vi "Histogram Main.vi"() -> ()   [LabVIEW 2012]
uses:
  Consumer Message.ctl
  <vilib>/Utility/file.llb/Write To Spreadsheet File (DBL).vi
panel:
  in  "signal":u16(ring) items=["uniform white", "uniform+uniform", "Gaussian white", "sine", "square"]
  in  "Snapshot":bool
  out "Histogram":cluster{"histogram":dbl[], "x axis":dbl[]}(graph)
  in  "bins":i32=20
  out "Consumer Shutdown?":bool
  out "Backlog":u8(slide) scale=0.0..100.0
  in  "Stop":bool
  # "Number of enqueued messages waiting to be processed"
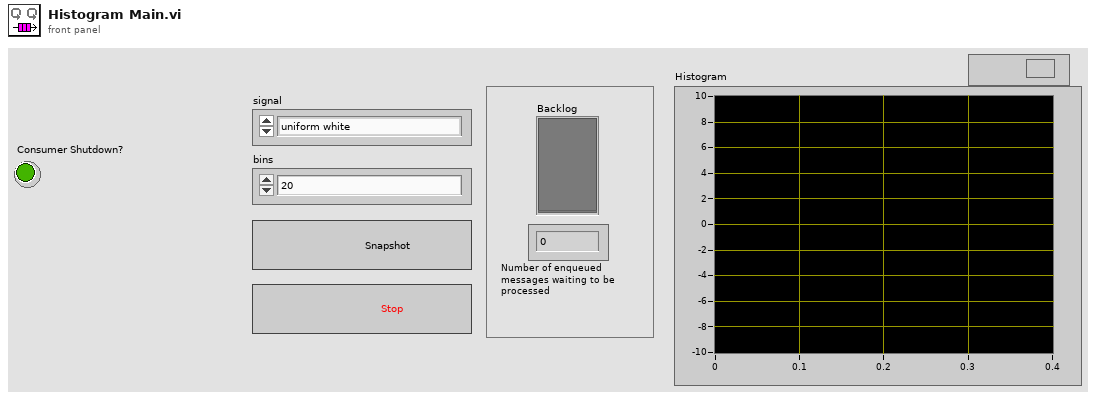
[diagram p1: front panel]
types:
  T1 = typedef "Consumer Message.ctl" = cluster{"Consumer State":string, "Boolean Data":bool, "Numeric Data":i32, "Signal":dbl[], "Error":errorcluster}
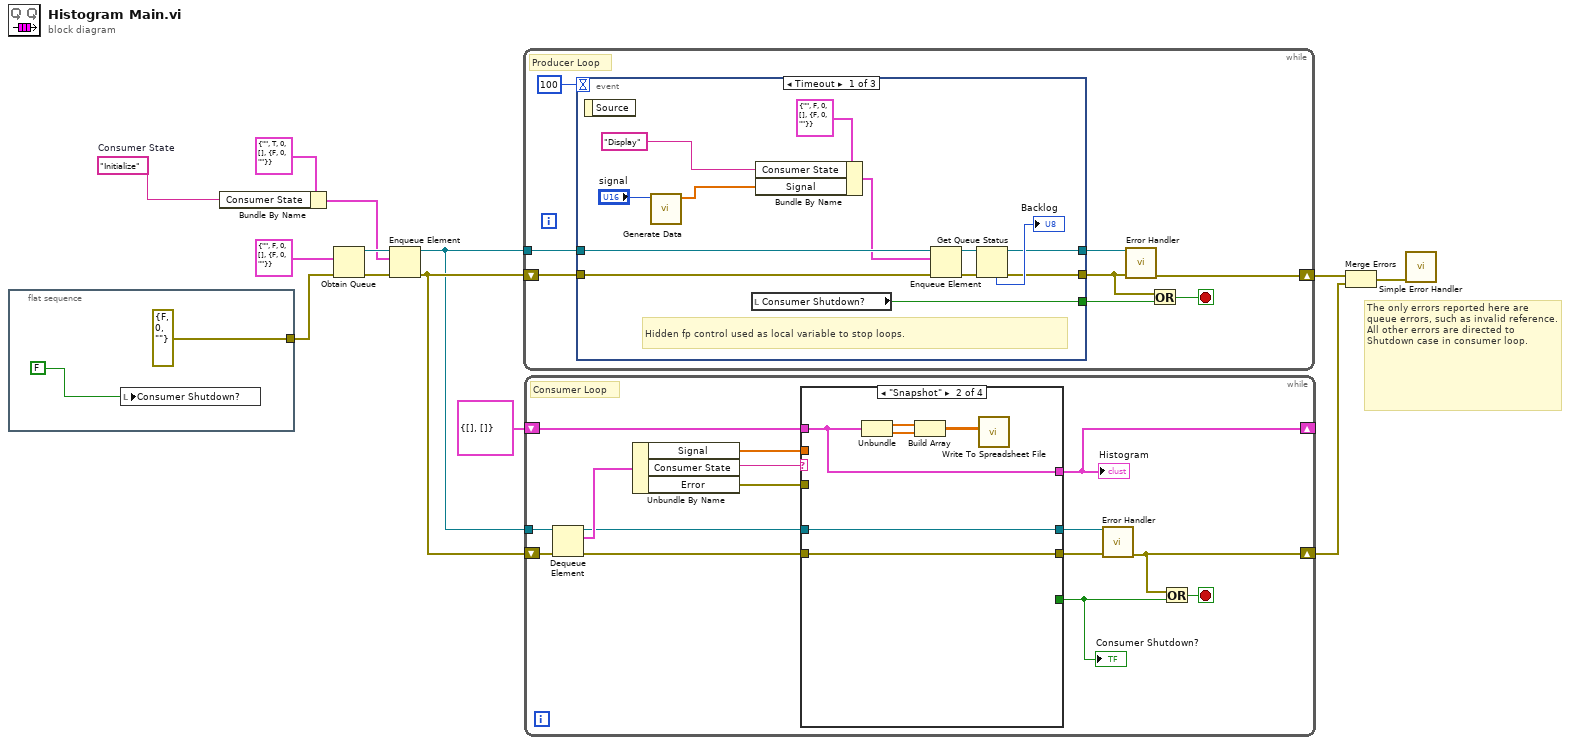
[diagram p0: block diagram]
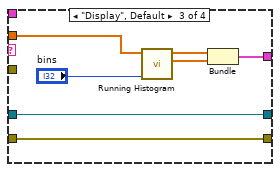
[diagram p3: hidden frame]
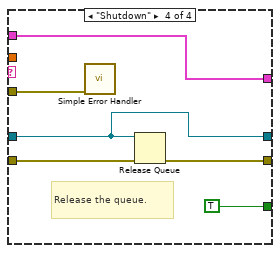
[diagram p4: hidden frame]
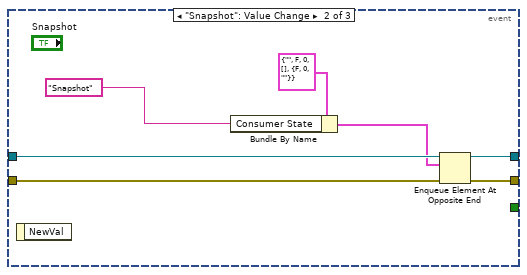
[diagram p5: hidden frame]
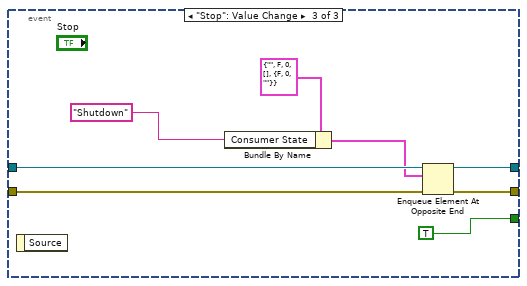
[diagram p6: hidden frame]
diagram:
  w5 = "Initialize"  # Consumer State
  # "The only errors reported here are queue errors, such as invalid reference.  All other errors are directed to Shutdown case in consumer loop."
  n1 = flat-sequence {
    tunnel: [errorcluster {"status"=FALSE, "code"=0, "source"=""} ("error in (no error)")] -> w8
    frame #0 {
      n2 = local write "Consumer Shutdown?"(FALSE ("Stop Loops (local)")) -> ()
    }
  }
  n3 = Bundle By Name(cluster=T1 {"Consumer State"="", "Boolean Data"=TRUE, "Numeric Data"=0, "Signal"=[], "Error"={"status"=FALSE, "code"=0, "source"=""}} ("Consumer Message"), "Consumer State"=w5) -> (w6:T1)
  n4 = Obtain Queue(element data type=T1 {"Consumer State"="", "Boolean Data"=FALSE, "Numeric Data"=0, "Signal"=[], "Error"={"status"=FALSE, "code"=0, "source"=""}}, error in (no error)=w8) -> (queue out=w10:refnum<queue>, error out=w13:errorcluster)  [unwired: 3 in, 1 out]
  n5 = Enqueue Element(queue=w10, element=w6, error in (no error)=w13) -> (queue out=w9:refnum<queue>, error out=w11:errorcluster)  [unwired: 1 in, 1 out]
  n6 = while {
    tunnel: w9 -> [w23]
    shift-right: [w16] -> w4
    shift-left: w11 -> [w22]
    stop <- w18 stop-if-true
    # "Producer Loop"
    n7 = event shown="[0] Timeout" {
      selector: _ -> [_ _ _]
      dyn-events: _ -> [_ _ _]
      timeout: 100 -> [_ _ _]
      tunnel: w23 -> [w34 w42 w51]
      tunnel: w22 -> [w30 w41 w49]
      tunnel: [w33 w43 w48] -> w17
      tunnel: [w36 _ TRUE] -> w19
      tunnel: [w32 w38 w47] -> w21
      event Timeout {
        # "Hidden fp control used as local variable to stop loops."
        n8 = event-data() -> ()  [unwired: 1 in, 1 out]
        n9 = call "Generate Data.vi"("signal"="signal") -> ("Y"=w26:dbl[])  [unwired: 9 in, 1 out]
        n10 = local read "Consumer Shutdown?"() -> (w36:bool)
        n11 = Bundle By Name(cluster=T1 {"Consumer State"="", "Boolean Data"=FALSE, "Numeric Data"=0, "Signal"=[], "Error"={"status"=FALSE, "code"=0, "source"=""}}, "Consumer State"="Display", "Signal"=w26) -> (w27:T1)
        n12 = Enqueue Element(queue=w34, element=w27, error in (no error)=w30) -> (queue out=w31:refnum<queue>, error out=w29:errorcluster)  [unwired: 1 in, 1 out]
        n13 = Get Queue Status(queue=w31, error in (no error)=w29) -> (queue out=w32:refnum<queue>, error out=w33:errorcluster, # elements in queue=→"Backlog":i32)  [unwired: 1 in, 5 out]
      }
      event "Snapshot": Value Change {
        n14 = event-data() -> ()  [unwired: 1 in, 1 out]
        n15 = Bundle By Name(cluster=T1 {"Consumer State"="", "Boolean Data"=FALSE, "Numeric Data"=0, "Signal"=[], "Error"={"status"=FALSE, "code"=0, "source"=""}}, "Consumer State"="Snapshot" ("String Data")) -> (w39:T1)
        n16 = Enqueue Element At Opposite End(queue=w42, element=w39, error in (no error)=w41) -> (queue out=w38:refnum<queue>, error out=w43:errorcluster)  [unwired: 1 in, 1 out]
      }
      event "Stop": Value Change {
        n17 = event-data() -> ()  [unwired: 1 in, 1 out]
        n18 = Bundle By Name(cluster=T1 {"Consumer State"="", "Boolean Data"=FALSE, "Numeric Data"=0, "Signal"=[], "Error"={"status"=FALSE, "code"=0, "source"=""}}, "Consumer State"="Shutdown") -> (w44:T1)
        n19 = Enqueue Element At Opposite End(queue=w51, element=w44, error in (no error)=w49) -> (queue out=w47:refnum<queue>, error out=w48:errorcluster)  [unwired: 1 in, 1 out]
      }
    }
    n20 = call "Error Handler.vi"("error in"=w17, "queue in"=w21) -> ("error out"=w16:errorcluster)  [unwired: 8 in, 1 out]
    n21 = Or(x=w17, y=w19) -> (x .or. y?=w18:bool)
  }
  n22 = while {
    tunnel: w9 -> [w66]
    shift-right: [w57] -> w3
    shift-left: w11 -> [w65]
    shift-right: [w54] -> _
    shift-left: cluster{"histogram":dbl[], "x axis":dbl[]} {"histogram"=[], "x axis"=[]} -> [w53]
    stop <- w58 stop-if-true
    # "Consumer Loop"
    n23 = Dequeue Element(queue=w66, error in (no error)=w65) -> (queue out=w56:refnum<queue>, element=w64:T1, error out=w55:errorcluster)  [unwired: 1 in, 1 out]
    n24 = Unbundle By Name(w64) -> ("Signal"=w52:dbl[], "Consumer State"=w63:string, "Error"=w60:errorcluster)
    n25 = case shown="\"Snapshot\"" w63 {
      tunnel: [_ _ _ TRUE] -> w59
      tunnel: w55 -> [w68 w74 w81 w87]
      tunnel: [w68 w74 w81 w86] -> w62
      tunnel: w56 -> [w69 w75 w82 w84]
      tunnel: [w69 w75 w82 w84] -> w61
      tunnel: w60 -> [_ _ _ w85]
      tunnel: [w67 w70 w77 w83] -> w54
      tunnel: w53 -> [w67 w70 _ w83]
      tunnel: w52 -> [_ _ w76 _]
      frame "Initialize" {
      }
      frame "Snapshot" {
        n26 = Unbundle(w70) -> ("histogram"=w73:dbl[], "x axis"=w72:dbl[])
        n27 = Build Array(w73, w72) -> (w71:dbl[][])
        n28 = call-poly <vilib>:"Write To Spreadsheet File.vi"("2D data"=w71) -> ()  [unwired: 7 in, 1 out]
      }
      frame "Display", Default {
        n29 = call "Running Histogram.vi"("bins"="bins", "input data"=w76) -> ("x axis"=w78:dbl[], "histogram"=w79:dbl[])  [unwired: 6 in, 2 out]
        n30 = Bundle("histogram"=w79, "x axis"=w78) -> (w77:cluster{"histogram":dbl[], "x axis":dbl[]})  [unwired: 1 in]
      }
      frame "Shutdown" {
        # "Release the queue."
        n31 = call <vilib>:"Simple Error Handler.vi"("error in (no error)"=w85) -> ()  [unwired: 4 in, 5 out]
        n32 = Release Queue(queue=w84, error in (no error)=w87) -> (error out=w86:errorcluster)  [unwired: 1 in, 2 out]
      }
    }
    "Consumer Shutdown?" <- w59
    "Histogram" <- w54
    n33 = call "Error Handler.vi"("error in"=w62, "queue in"=w61) -> ("error out"=w57:errorcluster)  [unwired: 8 in, 1 out]
    n34 = Or(x=w57, y=w59) -> (x .or. y?=w58:bool)
  }
  n35 = Merge Errors(w4, w3) -> (w2:errorcluster)
  n36 = call <vilib>:"Simple Error Handler.vi"("error in (no error)"=w2) -> ()  [unwired: 4 in, 5 out]
